vi "vision data fg.vi"(1 "Input":T1, 2 "Menu":T2) -> (0 "Output":T1)   [LabVIEW 2012]
uses:
  typedefs/fg_typedef.ctl
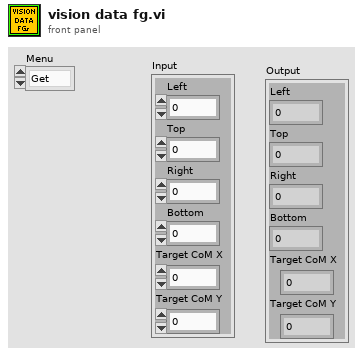
[diagram p1: front panel]
types:
  T1 = cluster{"Left":dbl, "Top":dbl, "Right":dbl, "Bottom":dbl, "Target CoM X":dbl, "Target CoM Y":dbl}
  T2 = typedef "fg_typedef.ctl" = enum16{"Get", "Set"}
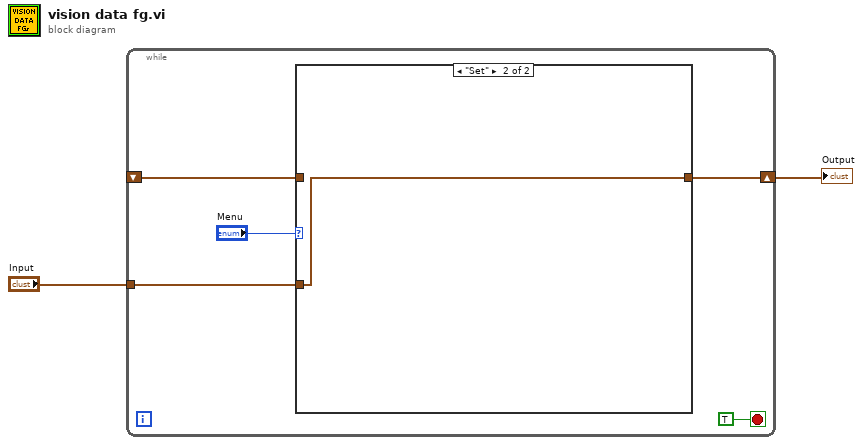
[diagram p0: block diagram]
diagram:
  n1 = while {
    shift-right: [w3] -> w1
    shift-left: _ -> [w5]
    tunnel: "Input" -> [w4]
    stop <- TRUE stop-if-true
    n2 = case shown="\"Set\"" "Menu" {
      tunnel: w5 -> [w8 _]
      tunnel: w4 -> [_ w9]
      tunnel: [w8 w9] -> w3
      frame "Get", Default {
      }
      frame "Set" {
      }
    }
  }
  "Output" <- w1
